vi "XLP80_Datalog_CheckLogSelect.vi"(8 "error in":errorcluster caption="error out") -> (0 "error OUT":errorcluster caption="error out")   [LabVIEW 2021]
doc: "Es wird der Dateiname überprüft und die erste Zeile des Files erzeugt (Spaltenbezeichnung). In der ersten Zeile stehen die Kanalnamen und die Zeit, in der zweiten Zeile stehen die Einheiten."
uses:
  XLP80_Datalog_TypeDefEnumLogselect.ctl
  XLP80_FGlob/XLP80_FGLob_TDefEnumCalcAnalogItems.ctl
panel:
  in  "LogSelect":u16(ring)=1 items=["SMART.No.MaxCell [-]", "SMART.No.MinCell [-]", "SMART.U.S.AveCell [V]", "SMART.U.S.CVM [V]", "SMART.U.S.MaxCell [V]", "SMART.U.S.MinCell [V]"]
  out "x = y?":bool
  in  "CalculatedValues_Items":T1
  in  "LogSelect":T2
  # "Ring"
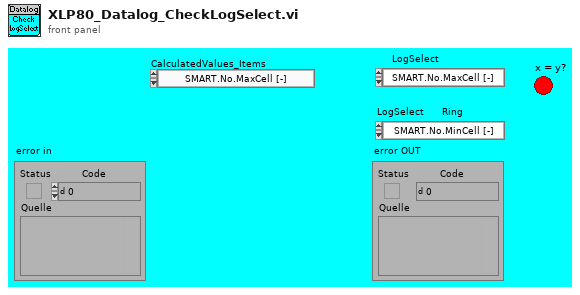
[diagram p1: front panel]
types:
  T1 = typedef "XLP80_FGLob_TDefEnumCalcAnalogItems.ctl" = enum8{"SMART.No.MaxCell [-]", "SMART.No.MinCell [-]", "SMART.U.S.AveCell [V]", "SMART.U.S.CVM [V]", "SMART.U.S.MaxCell [V]", "SMART.U.S.MinCell [V]"}
  T2 = typedef "XLP80_Datalog_TypeDefEnumLogselect.ctl" = enum16{"SMART.No.MaxCell [-]", "SMART.No.MinCell [-]", "SMART.U.S.AveCell [V]", "SMART.U.S.CVM [V]", "SMART.U.S.MaxCell [V]", "SMART.U.S.MinCell [V]"}
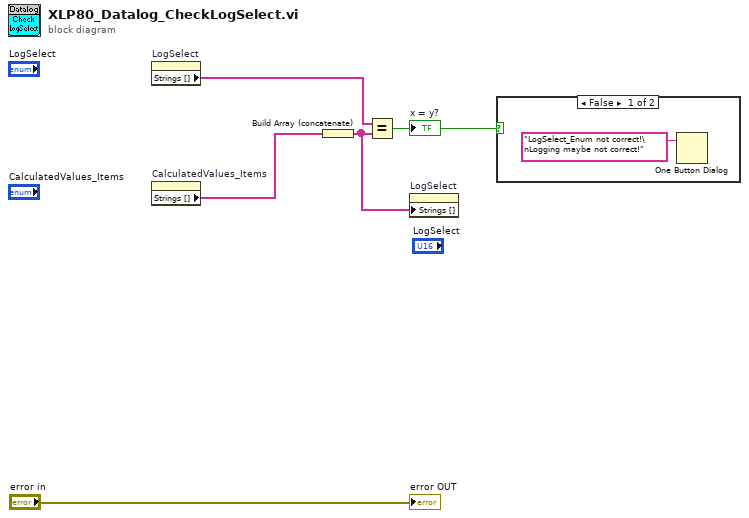
[diagram p0: block diagram]
diagram:
  n1 = property on="LogSelect" class="Enum (strict)"() -> ("Strings []"=w3:string[])  [unwired: 2 in, 2 out]
  n2 = property on="CalculatedValues_Items" class="Enum (strict)"() -> ("Strings []"=w4:string[])  [unwired: 2 in, 2 out]
  n3 = Build Array (concatenate)(w4) -> (w2:string[])
  n4 = Equal?(x=w3, y=w2) -> (x = y?=w1:bool)
  "x = y?" <- w1
  n5 = property on="LogSelect" class="Ring (strict)"("Strings []"=w2) -> ()  [unwired: 2 in, 2 out]
  n6 = case shown="False" w1 {
    frame False {
      n7 = One Button Dialog(message="LogSelect_Enum not correct!\nLogging maybe not correct!") -> ()  [unwired: 1 in, 1 out]
    }
    frame True {
    }
  }
  "error OUT" <- "error in"
